vi "New Table From Document.vi"(8 "error in (no error)":errorcluster, 11 "xwpfTable in":refnum<class "xwpfTable.lvclass">) -> (0 "error out":errorcluster, 3 "xwpfTable out":refnum<class "xwpfTable.lvclass">)   [LabVIEW 2017, in "Word_Specific.lvlib" / "xwpfTable.lvclass"]
uses:
  xwpfTable.lvclass
  C:/Users/Neo/Desktop/Dev_Tools_BR/LabVIEW_NPOI/lib/NPOI 2.1.1/NPOI.OOXML.dll
  lib/NPOI 2.1.1/NPOI.OOXML.dll
  xwpfTable.lvclass/xwpfTable.ctl
panel:
  in  "Table Ref":refnum<k24>
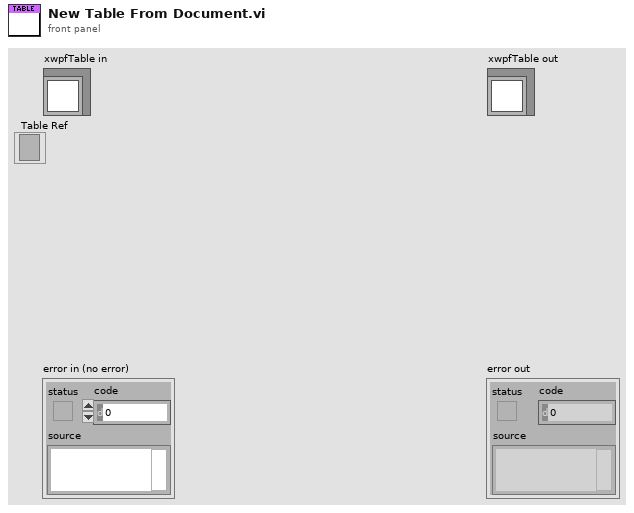
[diagram p1: front panel]
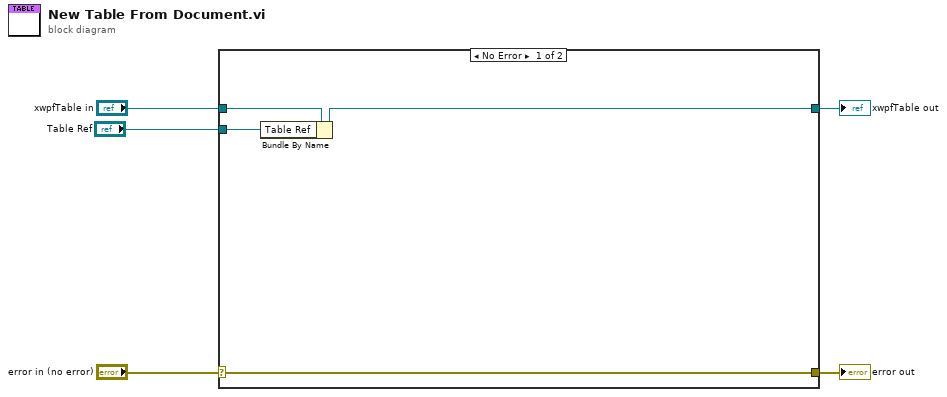
[diagram p0: block diagram]
diagram:
  n1 = case shown="No Error" "error in (no error)" {
    selector: "error in (no error)" -> [w8 w11]
    tunnel: [w8 w11] -> w4
    tunnel: [w7 w10] -> w2
    tunnel: "xwpfTable in" -> [w9 w10]
    tunnel: "Table Ref" -> [w6 _]
    frame No Error {
      n2 = Bundle By Name(cluster=w9, "Table Ref"=w6) -> (w7:refnum<class "xwpfTable.lvclass">)
    }
    frame Error {
    }
  }
  "error out" <- w4
  "xwpfTable out" <- w2
